vi "Get Fetch Type.vi"(8 "error in (no error)":errorcluster, 11 "Skyworks - 2G PVT in":refnum<class "Skyworks - PVT.lvclass">) -> (0 "error out":errorcluster, 3 "Skyworks - 2G PVT out":refnum<class "Skyworks - PVT.lvclass">)   [LabVIEW 2018, in "Skyworks PVT.lvlib" / "Skyworks - PVT.lvclass"]
uses:
  Skyworks - PVT.lvclass
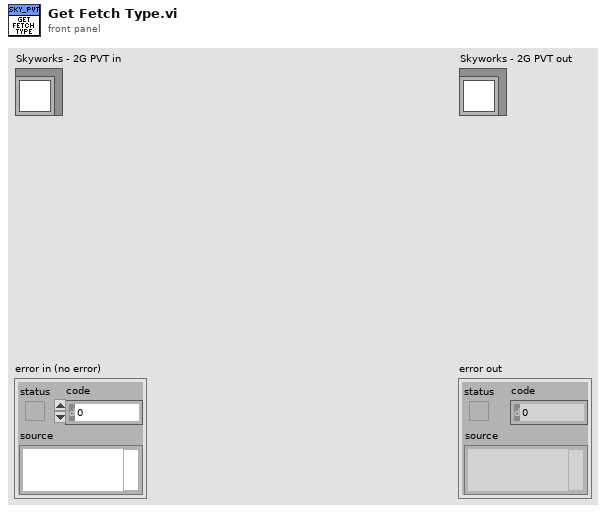
[diagram p1: front panel]
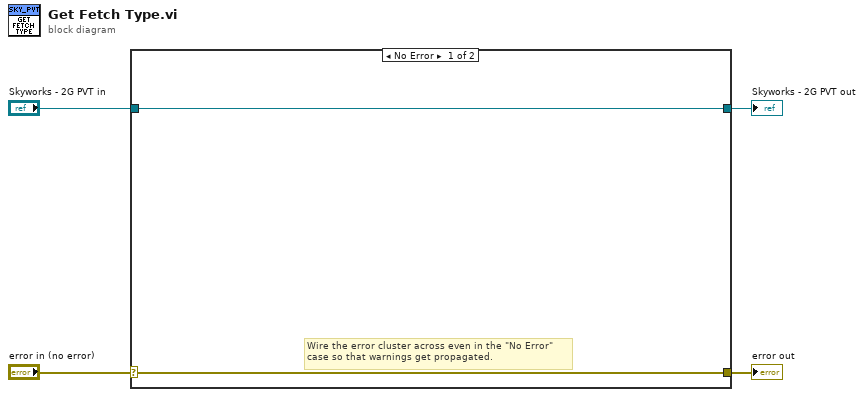
[diagram p0: block diagram]
diagram:
  n1 = case shown="No Error" "error in (no error)" {
    selector: "error in (no error)" -> [w5 w8]
    tunnel: [w5 w8] -> w3
    tunnel: [w6 w7] -> w1
    tunnel: "Skyworks - 2G PVT in" -> [w6 w7]
    frame No Error {
      # "Wire the error cluster across even in the \"No Error\"\ncase so that warnings get propagated."
    }
    frame Error {
    }
  }
  "error out" <- w3
  "Skyworks - 2G PVT out" <- w1
